vi "E7_20.vi"(4 "error in":T13, 7 "Command":T14) -> (0 "error out":T13, 3 "Response":T11)   [LabVIEW 2018]
uses:
  MOKO_LabViewLibrary/MokoLowLevel/MokoLowLovelControl/MLLC_Command.ctl
  MOKO_LabViewLibrary/MokoLowLevel/MokoLowLovelControl/MLLC_Error.ctl
  MOKO_LabViewLibrary/MokoLowLevel/MokoLowLovelControl/MLLC_Mode.ctl
  MOKO_LabViewLibrary/MokoLowLevel/MokoLowLovelControl/MLLC_Response.ctl
  MOKO_LabViewLibrary/MokoLowLevel/MokoLowLovelControl/MLLC_DriverName.ctl
  MOKO_LabViewLibrary/MokoLowLevel/MokoLowLovelControl/MLLC_ResponseInit.ctl
  MOKO_LabViewLibrary/MokoLowLevel/MokoLowLovelControl/MLLC_ErrorCode.ctl
  MOKO_LabViewLibrary/MokoLowLevel/MokoLowLovelControl/MLLC_Request.ctl
  MOKO_LabViewLibrary/MokoLowLevel/MokoLowLovelControl/MLLC_ConnectCluster.ctl
  MOKO_LabViewLibrary/MokoLowLevel/MokoLowLovelControl/MLLC_InterfaceType.ctl
  MOKO_LabViewLibrary/MokoLowLevel/MokoLowLovelControl/MLLC_OpenedSession.ctl
  MOKO_LabViewLibrary/MokoLowLevel/MokoLowLovelControl/MLLC_InterfaceSettings.ctl
  MOKO_LabViewLibrary/MokoLowLevel/MokoLowLovelControl/MLLC_InterfaceKind.ctl
  MOKO_LabViewLibrary/MokoLowLevel/MokoLowLovelControl/MLLC_Rs232Settings.ctl
panel:
  in  "Settings":T7={"Data"={"Connect"={"InterfaceType"=enum."VISA", "OpenedSession"="", "InterfaceSettings"={"Interface"=enum."RS232", "EOS 4 read"=enum."LF (\\n)", "EOS 4 write"=enum."LF (\\n)", "TMO, ms"=10000, "Sett"=variant(cluster{"Baud Rate":u32, "Data Bits":u16, "Parity":u16, "Stop Bits":u16, "Flow Control":u16, "Eho":bool} {"Baud Rate"=75, "Data Bits"=0, "Parity"=0, "Stop Bits"=0, "Flow Control"=0, "Eho"=FALSE})}}, "Function"=enum."VDC", "Delay, ms"=100}, "Saved Data"=variant}
  in  "Request":T8
  in  "Error Code":T6=5422
  in  "ResponseInit":T9="Є"
  in  "Driver Name":T10="E7_20"
  in  "Mode":T12=enum."Check"
  # "E7-20"
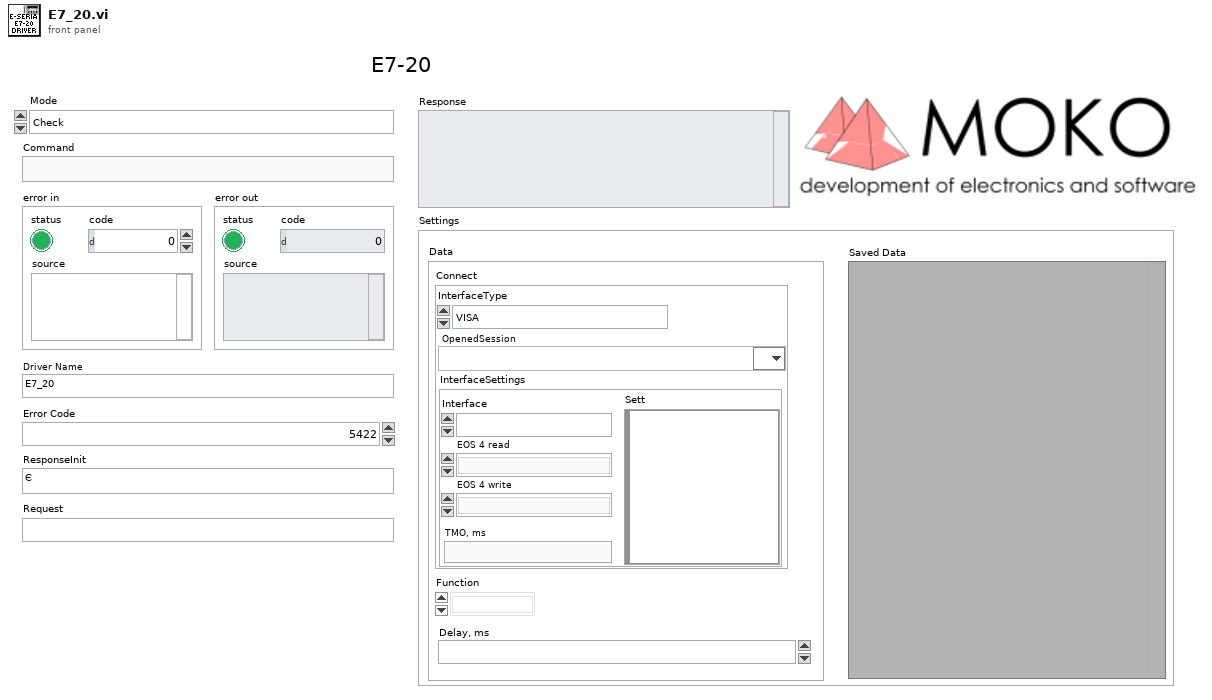
[diagram p1: front panel]
types:
  T1 = typedef "MLLC_ConnectCluster.ctl" = cluster{"InterfaceType":T2, "OpenedSession":T3, "InterfaceSettings":T4}
  T2 = typedef "MLLC_InterfaceType.ctl" = enum16{"VISA", "Prologix USB-GPIB"}
  T3 = typedef "MLLC_OpenedSession.ctl" = refnum<visa-resource-name>
  T4 = typedef "MLLC_InterfaceSettings.ctl" = cluster{"Interface":T5, "EOS 4 read":enum16{"Default (=EOS 4 write)", "CR (\\r)", "LF (\\n)", "None"}, "EOS 4 write":enum16{"CR+LF (\\r\\n)", "CR (\\r)", "LF (\\n)", "None"}, "TMO, ms":i32, "Sett":variant}
  T5 = typedef "MLLC_InterfaceKind.ctl" = enum16{"RS232", "GPIB", "USB", "Ethernet", "another"}
  T6 = typedef "MLLC_ErrorCode.ctl" = u32
  T7 = cluster{"Data":cluster{"Connect":T1, "Function":enum16{"F", "T", "R4", "R", "IAC", "IDC", "VAC", "VDC"}, "Delay, ms":T6}, "Saved Data":variant}
  T8 = typedef "MLLC_Request.ctl" = string
  T9 = typedef "MLLC_ResponseInit.ctl" = string
  T10 = typedef "MLLC_DriverName.ctl" = string
  T11 = typedef "MLLC_Response.ctl" = string
  T12 = typedef "MLLC_Mode.ctl" = enum16{"get", "set", "close", "Init", "Check"}
  T13 = typedef "MLLC_Error.ctl" = errorcluster
  T14 = typedef "MLLC_Command.ctl" = string
  T15 = cluster{"Connect":T1, "Function":enum16{"F", "T", "R4", "R", "IAC", "IDC", "VAC", "VDC"}, "Delay, ms":T6}
  T16 = typedef "MLLC_Rs232Settings.ctl" = cluster{"Baud Rate":u32, "Data Bits":u16, "Parity":u16, "Stop Bits":u16, "Flow Control":u16, "Eho":bool, "Address":dbl}
  T17 = enum16{"F", "T", "R4", "R", "IAC", "IDC", "VAC", "VDC"}
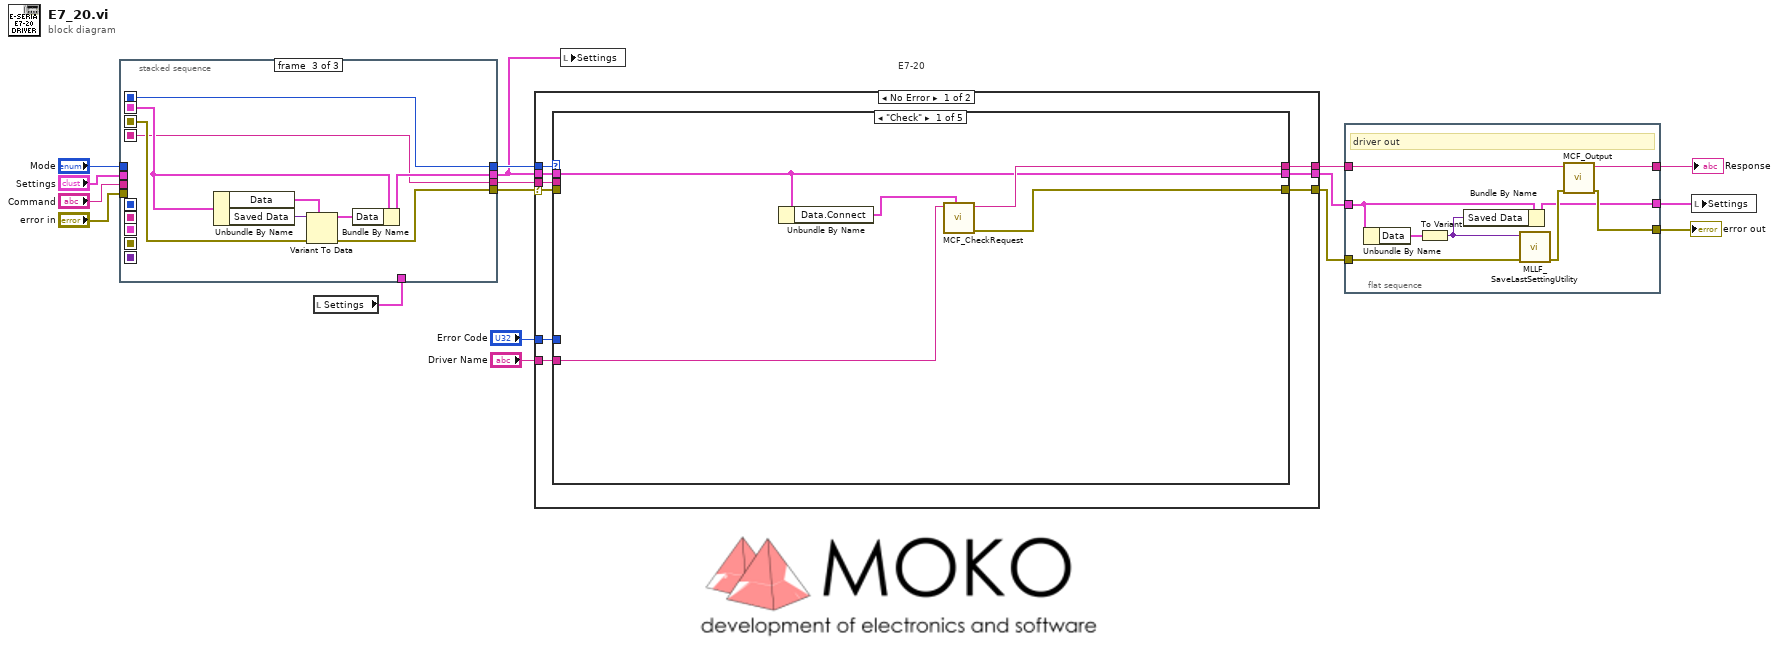
[diagram p0: block diagram]
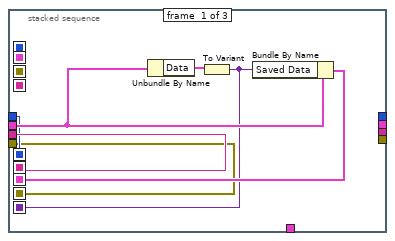
[diagram p2: hidden frame]
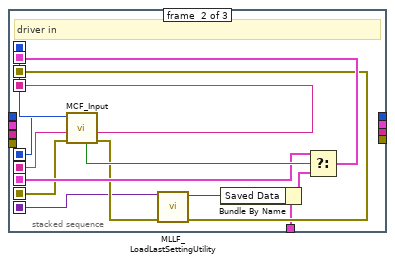
[diagram p3: hidden frame]
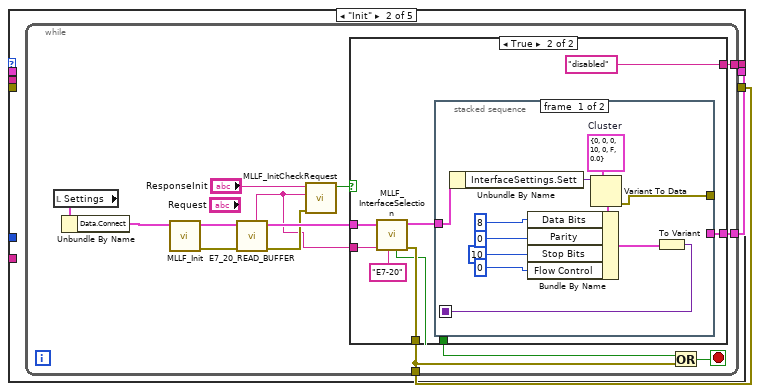
[diagram p4: hidden frame]
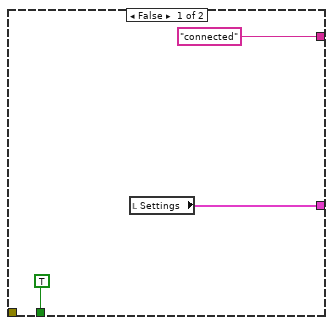
[diagram p5: hidden frame]
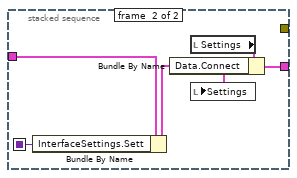
[diagram p6: hidden frame]
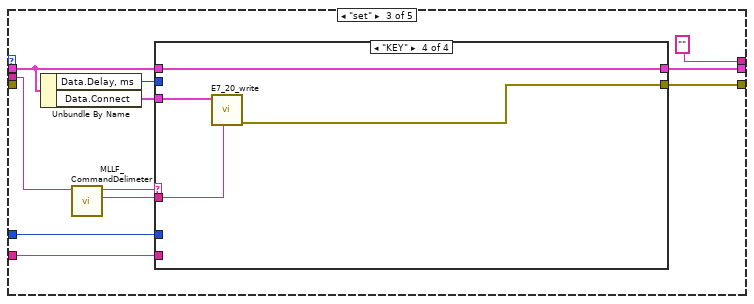
[diagram p7: hidden frame]
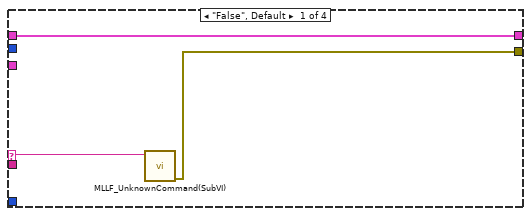
[diagram p8: hidden frame]
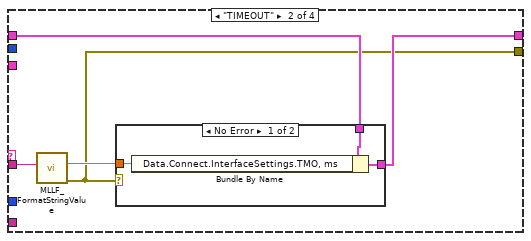
[diagram p9: hidden frame]
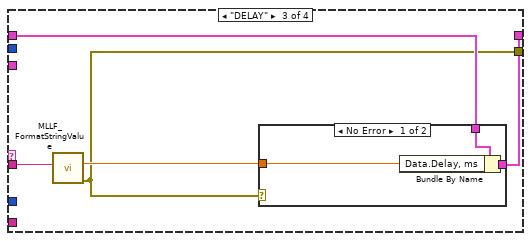
[diagram p11: hidden frame]
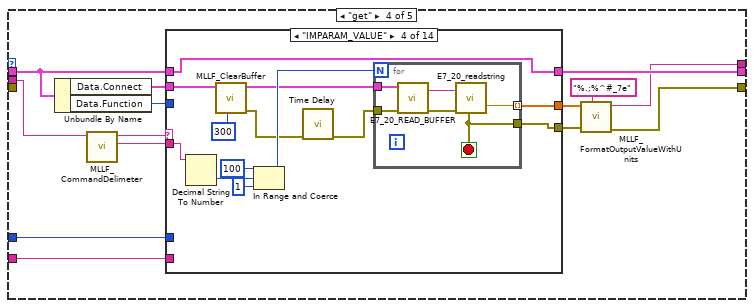
[diagram p13: hidden frame]
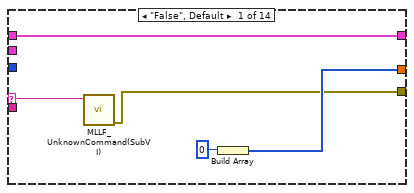
[diagram p14: hidden frame]
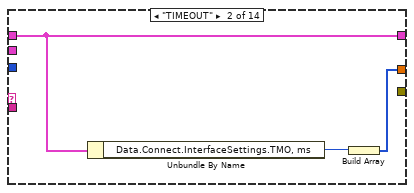
[diagram p15: hidden frame]
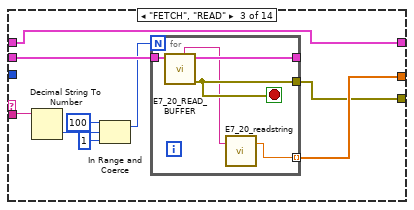
[diagram p16: hidden frame]
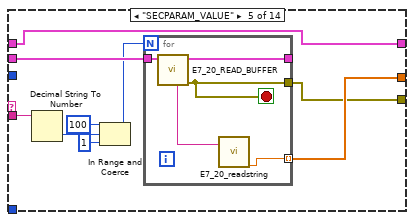
[diagram p17: hidden frame]
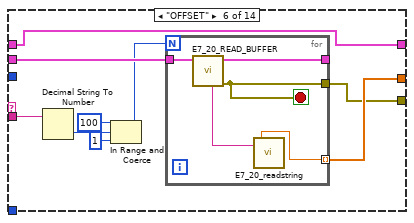
[diagram p18: hidden frame]
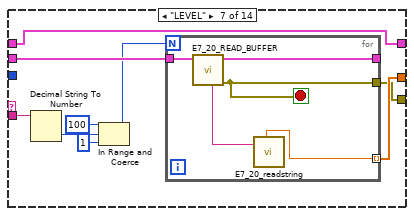
[diagram p19: hidden frame]
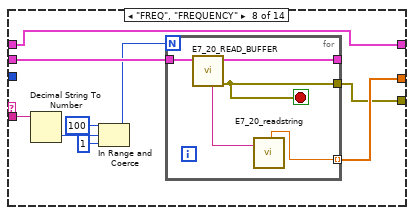
[diagram p20: hidden frame]
diagram:
  # "E7-20"
  n1 = local read "Settings"() -> (w7:T7)
  n2 = stacked-sequence {
    seq-local: [w20 _ _] -> [_ w36 _]
    seq-local: [w19 _ _] -> [_ w37 _]
    seq-local: [w22 _ _] -> [_ w32 _]
    seq-local: [w18 _ _] -> [_ w31 _]
    seq-local: [w21 _ _] -> [_ w27 _]
    seq-local: [_ w28 _] -> [_ _ w44]
    seq-local: [_ w38 _] -> [_ _ w41]
    seq-local: [_ w35 _] -> [_ _ w40]
    seq-local: [_ w34 _] -> [_ _ w45]
    tunnel: "Command" -> [w20 _ _]
    tunnel: "Mode" -> [w19 _ _]
    tunnel: "error in" -> [w18 _ _]
    tunnel: "Settings" -> [w23 _ _]
    tunnel: w7 -> [_ w26 _]
    tunnel: [_ _ w40] -> w9
    tunnel: [_ _ w43] -> w10
    tunnel: [_ _ w42] -> w8
    tunnel: [_ _ w41] -> w11
    frame #0 {
      n3 = Unbundle By Name(w23) -> ("Data"=w24:T15)
      n4 = To Variant(anything=w24) -> (Variant=w21:variant)
      n5 = Bundle By Name(cluster=w23, "Saved Data"=w21) -> (w22:T7)
    }
    frame #1 {
      # "driver in"
      n6 = call "MCF_Input.vi"("Error In"=w31, "Command in"=w36, "Mode in"=w37) -> ("Error Out"=w30:errorcluster, "Command out"=w35:string, "Mode out"=w38:T12, "Boolean"=w33:bool)  [unwired: 5 in]
      n7 = call "MLLF_LoadLastSettingUtility.vi"("Error In"=w30, "Save data in"=w27) -> ("Error Out"=w28:errorcluster, "Save data out"=w25:variant)  [unwired: 8 in]
      n8 = Bundle By Name(cluster=w26, "Saved Data"=w25) -> (w29:T7)
      n9 = Select(t=w32, s=w33, f=w29) -> (s? t:f=w34:T7)
    }
    frame #2 {
      n10 = Unbundle By Name(w45) -> ("Data"=w46:T15, "Saved Data"=w39:variant)
      n11 = Variant To Data(error in=w44, type=w46, Variant=w39) -> (data=w47:T15, error out=w42:errorcluster)
      n12 = Bundle By Name(cluster=w45, "Data"=w47) -> (w43:T7)
    }
  }
  n13 = case shown="No Error" w8 {
    selector: w8 -> [w52 w342]
    tunnel: [w54 w342] -> w4
    tunnel: w11 -> [w56 _]
    tunnel: [w55 "" ("String")] -> w6
    tunnel: w9 -> [w53 _]
    tunnel: w10 -> [w49 w341]
    tunnel: "Error Code" -> [w51 _]
    tunnel: "Driver Name" -> [w50 _]
    tunnel: [w48 w341] -> w5
    frame No Error {
      n14 = case shown="\"Check\"" w56 {
        tunnel: [w61 w64 "" ("String") w142 _] -> w55
        tunnel: [w60 w62 w106 w143 w338] -> w54
        tunnel: w53 -> [_ _ w109 w146 _]
        tunnel: w52 -> [_ _ _ _ _]
        tunnel: w51 -> [_ _ w116 w153 _]
        tunnel: w50 -> [w59 _ w113 w152 _]
        tunnel: w49 -> [w58 _ w115 w155 w337]
        tunnel: [w58 w63 w114 w154 w337] -> w48
        frame "Check" {
          n15 = Unbundle By Name(w58) -> ("Data.Connect"=w57:T1)
          n16 = call "MCF_CheckRequest.vi"("Permanent data.Connect"=w57, "Driver Name"=w59) -> ("Error Out"=w60:errorcluster, "Output String"=w61:string)  [unwired: 8 in]
        }
        frame "Init" {
          n17 = while {
            tunnel: [w76] -> w62
            tunnel: [w67] -> w64
            tunnel: [w66] -> w63
            stop <- w75 stop-if-true
            n18 = local read "Settings"() -> (w78:T7)
            n19 = Unbundle By Name(w78) -> ("Data.Connect"=w77:T1)
            n20 = call "MLLF_Init.vi"("DriverConnect in"=w77) -> ("Error Out"=w71:errorcluster, "DriverConnect out"=w72:T1)  [unwired: 7 in]
            n21 = call "E7_20_READ_BUFFER.vi"("error in"=w71, "DriverConnect in"=w72) -> ("error out"=w69:T13, "DriverConnect out"=w73:T1, "String"=w65:string)  [unwired: 7 in]
            n22 = call "MLLF_InitCheckRequest.vi"("error in (no error)"=w69, "Answer"=w65, "Response Init"="ResponseInit") -> ("Design"=w68:bool)  [unwired: 5 in, 3 out]
            n23 = case shown="True" w68 {
              tunnel: [_ w87] -> w76
              tunnel: [TRUE w83] -> w74
              tunnel: w73 -> [_ w89]
              tunnel: ["connected" "disabled"] -> w67
              tunnel: [w79 w84] -> w66
              tunnel: w65 -> [_ w82]
              frame False {
                n24 = local read "Settings"() -> (w79:T7)
              }
              frame True {
                n25 = call "MLLF_InterfaceSelection.vi"("Driver Name"="E7-20" ("String"), "Answer:"=w82, "DriverConnect in"=w89) -> ("error out"=w87:T13, "DriverConnect out"=w88:T1, "stop init?"=w83:bool)  [unwired: 4 in, 2 out]
                n26 = stacked-sequence {
                  seq-local: [w92 _] -> [_ w104]
                  tunnel: w88 -> [w90 w102]
                  tunnel: [w98 _] -> _
                  tunnel: [_ w103] -> w84
                  frame #0 {
                    w99 = T16 {"Baud Rate"=0, "Data Bits"=0, "Parity"=0, "Stop Bits"=10, "Flow Control"=0, "Eho"=FALSE, "Address"=0.0}  # Cluster
                    n27 = Unbundle By Name(w90) -> ("InterfaceSettings.Sett"=w100:variant)
                    n28 = Variant To Data(type=w99, Variant=w100) -> (data=w97:T16, error out=w98:errorcluster)  [unwired: 1 in]
                    n29 = Bundle By Name(cluster=w97, "Data Bits"=u16 8 ("Serial Settings:Data Bits"), "Parity"=u16 0 ("Serial Settings:Parity"), "Stop Bits"=u16 10 ("Serial Settings:Stop Bits"), "Flow Control"=u16 0 ("Serial Settings:Flow Control")) -> (w91:T16)
                    n30 = To Variant(anything=w91) -> (Variant=w92:variant)
                  }
                  frame #1 {
                    n31 = Bundle By Name(cluster=w102, "InterfaceSettings.Sett"=w104) -> (w101:T1)
                    n32 = local read "Settings"() -> (w105:T7)
                    n33 = Bundle By Name(cluster=w105, "Data.Connect"=w101) -> (w103:T7)
                    n34 = local write "Settings"(w103) -> ()
                  }
                }
              }
            }
            n35 = Or(x=w74, y=w76) -> (x .or. y?=w75:bool)
          }
        }
        frame "set" {
          n36 = Unbundle By Name(w115) -> ("Data.Delay, ms"=w110:T6, "Data.Connect"=w111:T1)
          n37 = call "MLLF_CommandDelimeter.vi"("command with param"=w109) -> ("param 1"=w107:string, "command"=w108:string)  [unwired: 6 in, 3 out]
          n38 = case shown="\"KEY\"" w108 {
            selector: w108 -> [w118 _ _ _]
            tunnel: w107 -> [_ w122 w131 w140]
            tunnel: [w117 w120 w129 w139] -> w106
            tunnel: w116 -> [_ _ _ _]
            tunnel: w115 -> [w119 w123 w132 w141]
            tunnel: [w119 w124 w133 w141] -> w114
            tunnel: w111 -> [_ _ _ w138]
            tunnel: w113 -> [_ _ _ _]
            tunnel: w110 -> [_ _ _ _]
            frame "False", Default {
              n39 = call "MLLF_UnknownCommand(SubVI).vi"("Unknown command"=w118) -> ("error out"=w117:errorcluster)  [unwired: 10 in]
            }
            frame "TIMEOUT" {
              n40 = call "MLLF_FormatStringValue.vi"("String Value"=w122) -> ("error out"=w120:T13, "number"=w121:dbl)  [unwired: 8 in, 1 out]
              n41 = case shown="No Error" w120 {
                tunnel: [w127 w128] -> w124
                tunnel: w123 -> [w126 w128]
                tunnel: w121 -> [w125 _]
                frame No Error {
                  n42 = Bundle By Name(cluster=w126, "Data.Connect.InterfaceSettings.TMO, ms"=w125) -> (w127:T7)
                }
                frame Error {
                }
              }
            }
            frame "DELAY" {
              n43 = call "MLLF_FormatStringValue.vi"("String Value"=w131) -> ("error out"=w129:T13, "number"=w130:dbl)  [unwired: 8 in, 1 out]
              n44 = case shown="No Error" w129 {
                tunnel: [w136 w137] -> w133
                tunnel: w132 -> [w135 w137]
                tunnel: w130 -> [w134 _]
                frame No Error {
                  n45 = Bundle By Name(cluster=w135, "Data.Delay, ms"=w134) -> (w136:T7)
                }
                frame Error {
                }
              }
            }
            frame "KEY" {
              n46 = call "E7_20_write.vi"("Command"=w140, "DriverConnect in"=w138) -> ("error out"=w139:T13)  [unwired: 8 in, 1 out]
            }
          }
        }
        frame "get" {
          n47 = Unbundle By Name(w155) -> ("Data.Connect"=w149:T1, "Data.Function"=w147:T17)
          n48 = call "MLLF_CommandDelimeter.vi"("command with param"=w146) -> ("param 1"=w144:string, "command"=w145:string)  [unwired: 6 in, 3 out]
          n49 = case shown="\"IMPARAM_VALUE\"" w145 {
            selector: w145 -> [w157 _ _ _ _ _ _ _ _ _ _ _ _ _]
            tunnel: w144 -> [_ _ w164 w178 w197 w211 w225 w239 w253 w267 w281 w295 w309 w323]
            tunnel: [w156 _ w169 w188 w202 w216 w230 w244 w258 w272 w286 w300 w314 w328] -> w151
            tunnel: w153 -> [_ _ _ _ _ _ _ _ _ _ _ _ _ _]
            tunnel: [w160 w163 w172 w190 w205 w219 w233 w247 w261 w275 w289 w303 w317 w331] -> w154
            tunnel: w155 -> [w160 w163 w172 w190 w205 w219 w233 w247 w261 w275 w289 w303 w317 w331]
            tunnel: [w158 w161 w170 w189 w203 w217 w231 w245 w259 w273 w287 w301 w315 w329] -> w150
            tunnel: w149 -> [_ _ w171 w181 w204 w218 w232 w246 w260 w274 w288 w302 w316 w330]
            tunnel: w152 -> [_ _ _ _ _ _ _ _ _ _ _ _ _ _]
            tunnel: w147 -> [_ _ _ _ _ _ _ _ _ _ _ _ _ _]
            frame "False", Default {
              n50 = call "MLLF_UnknownCommand(SubVI).vi"("Unknown command"=w157) -> ("error out"=w156:errorcluster)  [unwired: 10 in]
              n51 = Build Array(0 ("TimeOut")) -> (w158:i32[])
            }
            frame "TIMEOUT" {
              n52 = Unbundle By Name(w163) -> ("Data.Connect.InterfaceSettings.TMO, ms"=w162:i32)
              n53 = Build Array(w162) -> (w161:i32[])
            }
            frame "FETCH", "READ" {
              n54 = Decimal String To Number(string=w164) -> (number=w168:i32)  [unwired: 2 in, 1 out]
              n55 = In Range and Coerce(upper limit=100, x=w168, lower limit=1) -> (coerced(x)=w165:i32)  [unwired: 1 out]
              n56 = for {
                N: w165 -> [_]
                tunnel: [w173] -> w170 mode=indexing
                tunnel: [w176] -> w169
                tunnel: [w177] -> _
                tunnel: w171 -> [w175]
                stop <- w176 stop-if-true
                n57 = call "E7_20_READ_BUFFER.vi"("DriverConnect in"=w175) -> ("error out"=w176:T13, "DriverConnect out"=w177:T1, "String"=w174:string)  [unwired: 8 in]
                n58 = call "E7_20_readstring.vi"("read buffer"=w174) -> ("CS"=w173:dbl)  [unwired: 6 in, 12 out]
              }
            }
            frame "IMPARAM_VALUE" {
              n59 = Decimal String To Number(string=w178) -> (number=w187:i32)  [unwired: 2 in, 1 out]
              n60 = call "MLLF_ClearBuffer.vi"("Timeout(default = 300 ms)"=u32 300 ("Timeout"), "DriverConnect in"=w181) -> ("Error Out"=w180:errorcluster, "DriverConnect out"=w182:T1)  [unwired: 6 in, 1 out]
              n61 = In Range and Coerce(upper limit=100, x=w187, lower limit=1) -> (coerced(x)=w184:i32)  [unwired: 1 out]
              n62 = call "Time Delay"("error in (no error)"=w180) -> ("error out"=w179:errorcluster)  [unwired: 10 in]
              n63 = for {
                N: w184 -> [_]
                tunnel: [w194] -> w189 mode=indexing
                tunnel: [w192] -> w188
                tunnel: w182 -> [w195]
                tunnel: w179 -> [w191]
                stop <- w192 stop-if-true
                n64 = call "E7_20_READ_BUFFER.vi"("error in"=w191, "DriverConnect in"=w195) -> ("error out"=w193:T13, "String"=w196:string)  [unwired: 7 in, 1 out]
                n65 = call "E7_20_readstring.vi"("read buffer"=w196, "Error In"=w193) -> ("Error Out"=w192:errorcluster, "ImParam_Value"=w194:dbl)  [unwired: 5 in, 11 out]
              }
            }
            frame "SECPARAM_VALUE" {
              n66 = Decimal String To Number(string=w197) -> (number=w201:i32)  [unwired: 2 in, 1 out]
              n67 = In Range and Coerce(upper limit=100, x=w201, lower limit=1) -> (coerced(x)=w198:i32)  [unwired: 1 out]
              n68 = for {
                N: w198 -> [_]
                tunnel: [w206] -> w203 mode=indexing
                tunnel: [w209] -> w202
                tunnel: [w210] -> _
                tunnel: w204 -> [w207]
                stop <- w209 stop-if-true
                n69 = call "E7_20_READ_BUFFER.vi"("DriverConnect in"=w207) -> ("error out"=w209:T13, "DriverConnect out"=w210:T1, "String"=w208:string)  [unwired: 8 in]
                n70 = call "E7_20_readstring.vi"("read buffer"=w208) -> ("SecParam_Value"=w206:dbl)  [unwired: 6 in, 12 out]
              }
            }
            frame "OFFSET" {
              n71 = Decimal String To Number(string=w211) -> (number=w215:i32)  [unwired: 2 in, 1 out]
              n72 = In Range and Coerce(upper limit=100, x=w215, lower limit=1) -> (coerced(x)=w212:i32)  [unwired: 1 out]
              n73 = for {
                N: w212 -> [_]
                tunnel: [w220] -> w217 mode=indexing
                tunnel: [w223] -> w216
                tunnel: [w224] -> _
                tunnel: w218 -> [w221]
                stop <- w223 stop-if-true
                n74 = call "E7_20_READ_BUFFER.vi"("DriverConnect in"=w221) -> ("error out"=w223:T13, "DriverConnect out"=w224:T1, "String"=w222:string)  [unwired: 8 in]
                n75 = call "E7_20_readstring.vi"("read buffer"=w222) -> ("Offset"=w220:dbl)  [unwired: 6 in, 12 out]
              }
            }
            frame "LEVEL" {
              n76 = Decimal String To Number(string=w225) -> (number=w229:i32)  [unwired: 2 in, 1 out]
              n77 = In Range and Coerce(upper limit=100, x=w229, lower limit=1) -> (coerced(x)=w226:i32)  [unwired: 1 out]
              n78 = for {
                N: w226 -> [_]
                tunnel: [w234] -> w231 mode=indexing
                tunnel: [w237] -> w230
                tunnel: [w238] -> _
                tunnel: w232 -> [w235]
                stop <- w237 stop-if-true
                n79 = call "E7_20_READ_BUFFER.vi"("DriverConnect in"=w235) -> ("error out"=w237:T13, "DriverConnect out"=w238:T1, "String"=w236:string)  [unwired: 8 in]
                n80 = call "E7_20_readstring.vi"("read buffer"=w236) -> ("Level"=w234:dbl)  [unwired: 6 in, 12 out]
              }
            }
            frame "FREQ", "FREQUENCY" {
              n81 = Decimal String To Number(string=w239) -> (number=w243:i32)  [unwired: 2 in, 1 out]
              n82 = In Range and Coerce(upper limit=100, x=w243, lower limit=1) -> (coerced(x)=w240:i32)  [unwired: 1 out]
              n83 = for {
                N: w240 -> [_]
                tunnel: [w248] -> w245 mode=indexing
                tunnel: [w251] -> w244
                tunnel: [w252] -> _
                tunnel: w246 -> [w249]
                stop <- w251 stop-if-true
                n84 = call "E7_20_READ_BUFFER.vi"("DriverConnect in"=w249) -> ("error out"=w251:T13, "DriverConnect out"=w252:T1, "String"=w250:string)  [unwired: 8 in]
                n85 = call "E7_20_readstring.vi"("read buffer"=w250) -> ("Frequency"=w248:dbl)  [unwired: 6 in, 12 out]
              }
            }
            frame "FLAGS" {
              n86 = Decimal String To Number(string=w253) -> (number=w257:i32)  [unwired: 2 in, 1 out]
              n87 = In Range and Coerce(upper limit=100, x=w257, lower limit=1) -> (coerced(x)=w254:i32)  [unwired: 1 out]
              n88 = for {
                N: w254 -> [_]
                tunnel: [w262] -> w259 mode=indexing
                tunnel: [w265] -> w258
                tunnel: [w266] -> _
                tunnel: w260 -> [w263]
                stop <- w265 stop-if-true
                n89 = call "E7_20_READ_BUFFER.vi"("DriverConnect in"=w263) -> ("error out"=w265:T13, "DriverConnect out"=w266:T1, "String"=w264:string)  [unwired: 8 in]
                n90 = call "E7_20_readstring.vi"("read buffer"=w264) -> ("FLAGS"=w262:dbl)  [unwired: 6 in, 12 out]
              }
            }
            frame "MODE" {
              n91 = Decimal String To Number(string=w267) -> (number=w271:i32)  [unwired: 2 in, 1 out]
              n92 = In Range and Coerce(upper limit=100, x=w271, lower limit=1) -> (coerced(x)=w268:i32)  [unwired: 1 out]
              n93 = for {
                N: w268 -> [_]
                tunnel: [w276] -> w273 mode=indexing
                tunnel: [w279] -> w272
                tunnel: [w280] -> _
                tunnel: w274 -> [w277]
                stop <- w279 stop-if-true
                n94 = call "E7_20_READ_BUFFER.vi"("DriverConnect in"=w277) -> ("error out"=w279:T13, "DriverConnect out"=w280:T1, "String"=w278:string)  [unwired: 8 in]
                n95 = call "E7_20_readstring.vi"("read buffer"=w278) -> ("Mode"=w276:dbl)  [unwired: 6 in, 12 out]
              }
            }
            frame "LIMIT" {
              n96 = Decimal String To Number(string=w281) -> (number=w285:i32)  [unwired: 2 in, 1 out]
              n97 = In Range and Coerce(upper limit=100, x=w285, lower limit=1) -> (coerced(x)=w282:i32)  [unwired: 1 out]
              n98 = for {
                N: w282 -> [_]
                tunnel: [w290] -> w287 mode=indexing
                tunnel: [w293] -> w286
                tunnel: [w294] -> _
                tunnel: w288 -> [w291]
                stop <- w293 stop-if-true
                n99 = call "E7_20_READ_BUFFER.vi"("DriverConnect in"=w291) -> ("error out"=w293:T13, "DriverConnect out"=w294:T1, "String"=w292:string)  [unwired: 8 in]
                n100 = call "E7_20_readstring.vi"("read buffer"=w292) -> ("Limit"=w290:dbl)  [unwired: 6 in, 12 out]
              }
            }
            frame "IMPARAM" {
              n101 = Decimal String To Number(string=w295) -> (number=w299:i32)  [unwired: 2 in, 1 out]
              n102 = In Range and Coerce(upper limit=100, x=w299, lower limit=1) -> (coerced(x)=w296:i32)  [unwired: 1 out]
              n103 = for {
                N: w296 -> [_]
                tunnel: [w304] -> w301 mode=indexing
                tunnel: [w307] -> w300
                tunnel: [w308] -> _
                tunnel: w302 -> [w305]
                stop <- w307 stop-if-true
                n104 = call "E7_20_READ_BUFFER.vi"("DriverConnect in"=w305) -> ("error out"=w307:T13, "DriverConnect out"=w308:T1, "String"=w306:string)  [unwired: 8 in]
                n105 = call "E7_20_readstring.vi"("read buffer"=w306) -> ("ImParam"=w304:dbl)  [unwired: 6 in, 12 out]
              }
            }
            frame "SECPARAM" {
              n106 = Decimal String To Number(string=w309) -> (number=w313:i32)  [unwired: 2 in, 1 out]
              n107 = In Range and Coerce(upper limit=100, x=w313, lower limit=1) -> (coerced(x)=w310:i32)  [unwired: 1 out]
              n108 = for {
                N: w310 -> [_]
                tunnel: [w318] -> w315 mode=indexing
                tunnel: [w321] -> w314
                tunnel: [w322] -> _
                tunnel: w316 -> [w319]
                stop <- w321 stop-if-true
                n109 = call "E7_20_READ_BUFFER.vi"("DriverConnect in"=w319) -> ("error out"=w321:T13, "DriverConnect out"=w322:T1, "String"=w320:string)  [unwired: 8 in]
                n110 = call "E7_20_readstring.vi"("read buffer"=w320) -> ("SecParam"=w318:dbl)  [unwired: 6 in, 12 out]
              }
            }
            frame "ONCHANGE" {
              n111 = Decimal String To Number(string=w323) -> (number=w327:i32)  [unwired: 2 in, 1 out]
              n112 = In Range and Coerce(upper limit=100, x=w327, lower limit=1) -> (coerced(x)=w324:i32)  [unwired: 1 out]
              n113 = for {
                N: w324 -> [_]
                tunnel: [w332] -> w329 mode=indexing
                tunnel: [w335] -> w328
                tunnel: [w336] -> _
                tunnel: w330 -> [w333]
                stop <- w335 stop-if-true
                n114 = call "E7_20_READ_BUFFER.vi"("DriverConnect in"=w333) -> ("error out"=w335:T13, "DriverConnect out"=w336:T1, "String"=w334:string)  [unwired: 8 in]
                n115 = call "E7_20_readstring.vi"("read buffer"=w334) -> ("OnChange"=w332:dbl)  [unwired: 6 in, 12 out]
              }
            }
          }
          n116 = call "MLLF_FormatOutputValueWithUnits.vi"("Format"="%.;%^#_7e" ("format string"), "error in"=w151, "ValuesIn"=w150) -> ("error out"=w143:T13, "Result string"=w142:T14)  [unwired: 7 in]
        }
        frame "close" {
          n117 = Unbundle By Name(w337) -> ("Data.Connect.OpenedSession"=w339:T3)
          n118 = VISA Close(VISA resource name=w339) -> (error out=w338:errorcluster)  [unwired: 1 in]
        }
      }
    }
    frame Error {
    }
  }
  n119 = local write "Settings"(w10) -> ()
  n120 = flat-sequence {
    tunnel: [w351] -> w3
    tunnel: [w350] -> w1
    tunnel: w6 -> [w349]
    tunnel: w4 -> [w348]
    tunnel: w5 -> [w344]
    tunnel: [w346] -> w2
    frame #0 {
      # "driver out"
      n121 = Unbundle By Name(w344) -> ("Data"=w343:T15)
      n122 = To Variant(anything=w343) -> (Variant=w345:variant)
      n123 = Bundle By Name(cluster=w344, "Saved Data"=w345) -> (w346:T7)
      n124 = call "MLLF_SaveLastSettingUtility.vi"("error in"=w348, "Saved Data"=w345) -> ("error out"=w347:T13)  [unwired: 8 in, 1 out]
      n125 = call "MCF_Output.vi"("Error In"=w347, "Input"=w349) -> ("Error Out"=w350:errorcluster, "Output"=w351:string)  [unwired: 8 in]
    }
  }
  n126 = local write "Settings"(w2) -> ()
  "error out" <- w1
  "Response" <- w3
